vi "baselineparammaker.vi"(9 "weight <1":dbl, 10 "x":dbl[](array[numeric]), 11 "PEAKPOS ARRAY":cluster{"MIN":dbl, "MAX":dbl}[](array[cluster])) -> (3 "weight array":dbl[](array[numeric]))   [LabVIEW 2020]
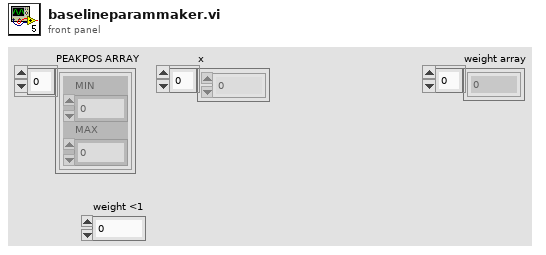
[diagram p1: front panel]
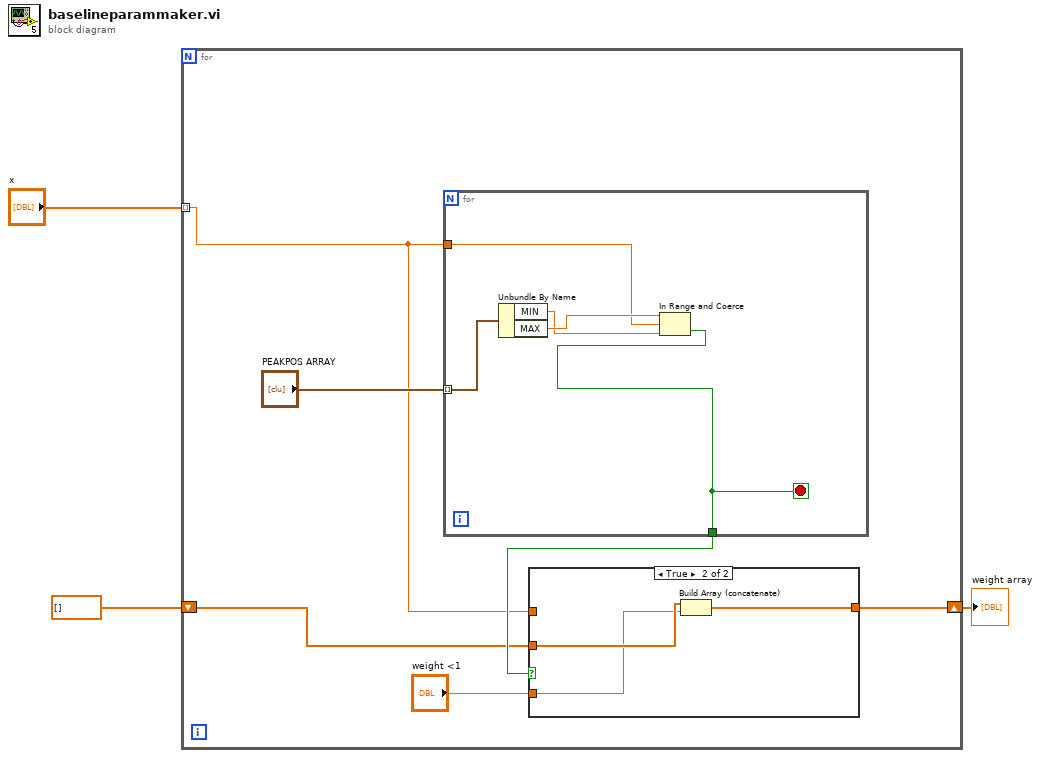
[diagram p0: block diagram]
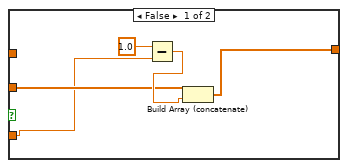
[diagram p2: hidden frame]
diagram:
  n1 = for {
    tunnel: "x" -> [w7] mode=indexing
    shift-right: [w5] -> w1
    shift-left: dbl[] [] ("weight array") -> [w6]
    n2 = for {
      tunnel: "PEAKPOS ARRAY" -> [w22] mode=indexing
      tunnel: w7 -> [w19]
      tunnel: [w18] -> w8
      stop <- w18 stop-if-true
      n3 = Unbundle By Name(w22) -> ("MIN"=w20:dbl, "MAX"=w21:dbl)
      n4 = In Range and Coerce(upper limit=w21, x=w19, lower limit=w20) -> (In Range?=w18:bool)  [unwired: 1 out]
    }
    n5 = case shown="True" w8 {
      tunnel: w7 -> [_ _]
      tunnel: w6 -> [w12 w17]
      tunnel: [w11 w16] -> w5
      tunnel: "weight <1" -> [w10 w15]
      frame False {
        n6 = Subtract(x=1.0, y=w10) -> (x-y=w13:dbl)
        n7 = Build Array (concatenate)(w12, w13) -> (w11:dbl[])
      }
      frame True {
        n8 = Build Array (concatenate)(w17, w15) -> (w16:dbl[])
      }
    }
  }
  "weight array" <- w1
